vi "RenameLayoutDialog.vi"(10 "Strings []":string[](array[string]), 11 "Change Layout Name:":string) -> (2 "New Layout name":string, 3 "Cancelled?":bool)   [LabVIEW 2013]
panel:
  in  "Cancel Button":bool
  in  "OK Button":bool
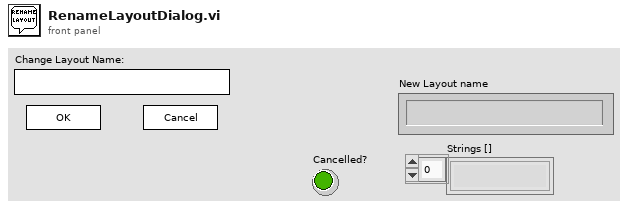
[diagram p1: front panel]
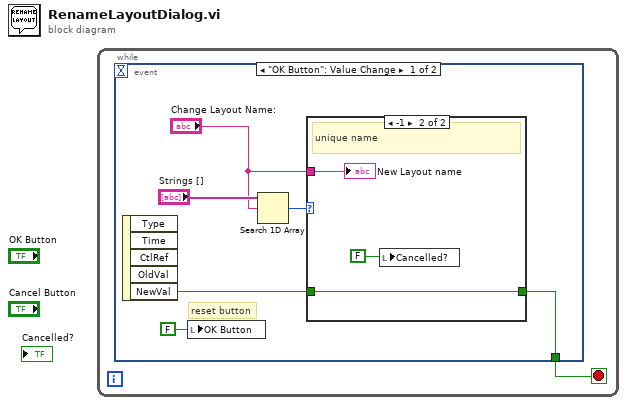
[diagram p0: block diagram]
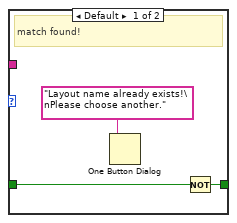
[diagram p2: hidden frame]
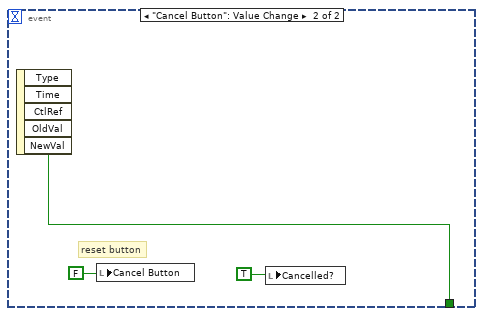
[diagram p3: hidden frame]
diagram:
  n1 = while {
    stop <- w1 stop-if-true
    n2 = event shown="[0] \"OK Button\": Value Change" {
      selector: _ -> [_ _]
      dyn-events: _ -> [_ _]
      timeout: _ -> [_ _]
      tunnel: [w6 w15] -> w1
      event "OK Button": Value Change {
        # "reset button"
        n3 = event-data() -> ("NewVal"=w5:bool)  [unwired: 1 in, 4 out]
        n4 = local write "OK Button"(FALSE) -> ()
        n5 = Search 1D Array(1D array="Strings []", element="Change Layout Name:") -> (index of element=w7:i32)  [unwired: 1 in]
        n6 = case shown="-1" w7 {
          tunnel: "Change Layout Name:" -> [_ w12]
          tunnel: w5 -> [w8 w11]
          tunnel: [w10 w11] -> w6
          frame Default {
            # "match found!"
            n7 = One Button Dialog(message="Layout name already exists!\nPlease choose another.") -> ()  [unwired: 1 in, 1 out]
            n8 = Not(x=w8) -> (.not. x?=w10:bool)
          }
          frame -1 {
            # "unique name"
            n9 = local write "Cancelled?"(FALSE) -> ()
            "New Layout name" <- w12
          }
        }
      }
      event "Cancel Button": Value Change {
        # "reset button"
        n10 = event-data() -> ("NewVal"=w15:bool)  [unwired: 1 in, 4 out]
        n11 = local write "Cancel Button"(FALSE) -> ()
        n12 = local write "Cancelled?"(TRUE) -> ()
      }
    }
  }
